vi "4017_18_get_rdg.vi"(4 "Channel Name":string, 7 "Address":T1) -> (1 "Reading":dbl format="%.3f", 3 "Comment":string)   [LabVIEW 2018]
uses:
  ADAM Client/Sub VIs/ADAM Controls/Address.ctl
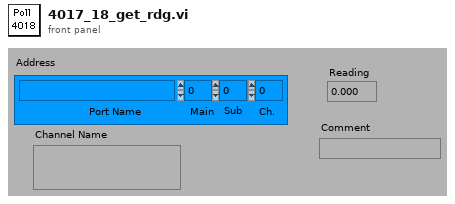
[diagram p1: front panel]
types:
  T1 = typedef "Address.ctl" = cluster{"Main":i32, "Ch.":i32, "Sub":i32, "Port Name":string}
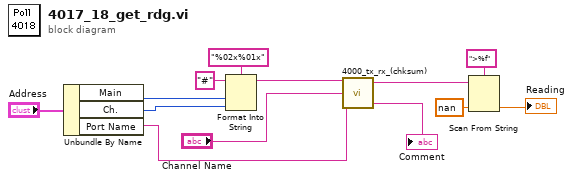
[diagram p0: block diagram]
diagram:
  n1 = Unbundle By Name("Address") -> ("Main"=w3:i32, "Ch."=w2:i32, "Port Name"=w1:string)
  n2 = Format Into String(format string="%02x%01x", initial string="#", w3, w2) -> (resulting string=w11:string)  [unwired: 1 in, 1 out]
  n3 = call "4000_tx_rx_(chksum).vi"("Write String"=w11, "Channel Name"="Channel Name", "Port Name"=w1) -> ("Read"=w9:string, "Comment out"=→"Comment":string)  [unwired: 2 in, 1 out]
  n4 = Scan From String(format string=">%f", input string=w9, default 1=nan ("Reading")) -> (output 1=→"Reading":dbl)  [unwired: 2 in, 3 out]
